vi "close game pad.vi"(8 "error in (no error)":errorcluster, 11 "Hardware Game Pad Interface in":refnum<class "Hardware Game Pad Interface.lvclass">) -> (0 "error out":errorcluster, 3 "Hardware Game Pad Interface out":refnum<class "Hardware Game Pad Interface.lvclass">)   [LabVIEW 2017, in "Hardware Game Pad Interface.lvclass"]
uses:
  Hardware Game Pad Interface.lvclass
  Hardware Game Pad Interface.lvclass/Hardware Game Pad Interface.ctl
  <vilib>/Utility/inputDevices.llb/closeJoystick.vi
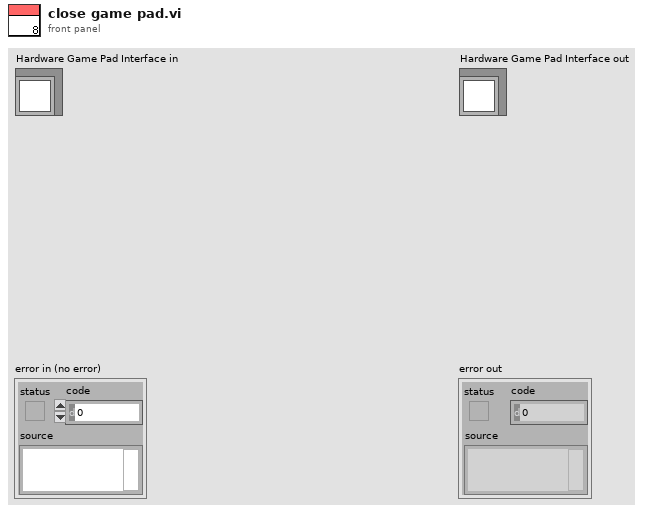
[diagram p1: front panel]
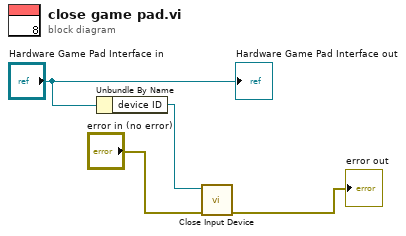
[diagram p0: block diagram]
diagram:
  n1 = Unbundle By Name("Hardware Game Pad Interface in") -> ("device ID"=w1:refnum<k1>)
  n2 = call-poly <vilib>:"Close Input Device.vi"("error in (no error)"="error in (no error)", "device ID"=w1) -> ("error out"=→"error out":errorcluster)  [unwired: 8 in]
  "Hardware Game Pad Interface out" <- "Hardware Game Pad Interface in"
